vi "GetKingPosition.vi"(10 "Color":T1, 11 "Input Squares":T2[][](array[typedef])) -> (3 "Position":i32[](array[numeric]))   [LabVIEW 2019]
doc: "This VI searches chessboard in case of finding particular pieces"
uses:
  #typedef_SquareType.ctl
  #typedef_Color.ctl
  #typedef_Piece.ctl
  #typedef_PieceType.ctl
panel:
  out "?":u16[][](array[ring])
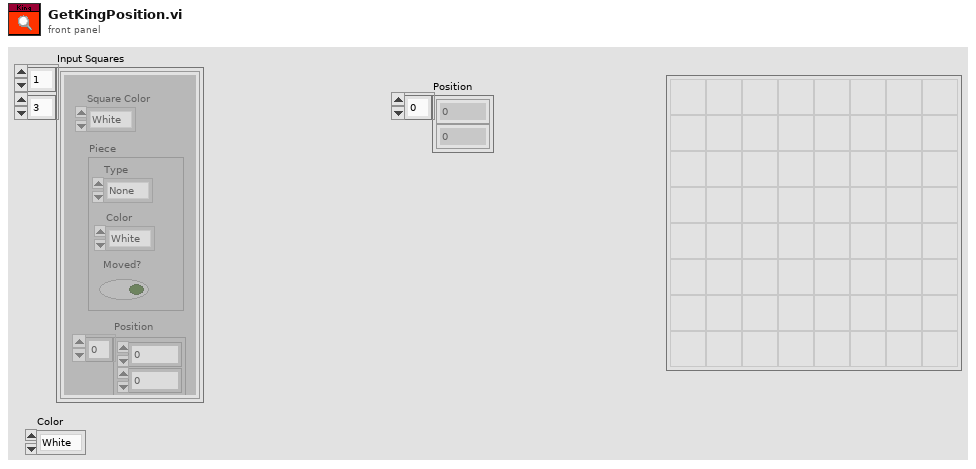
[diagram p1: front panel]
types:
  T1 = typedef "#typedef_Color.ctl" = enum16{"White", "Black"}
  T2 = typedef "#typedef_SquareType.ctl" = cluster{"Square Color":T1, "Position":i32[], "Piece":T3}
  T3 = typedef "#typedef_Piece.ctl" = cluster{"Type":T4, "Color":T1, "Moved?":bool}
  T4 = typedef "#typedef_PieceType.ctl" = enum16{"None", "Pawn", "Knight", "Bishop", "Rook", "Queen", "King"}
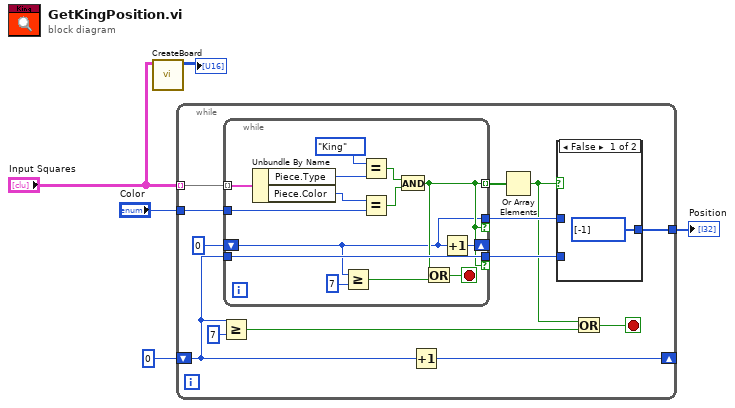
[diagram p0: block diagram]
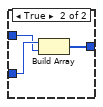
[diagram p2: hidden frame]
diagram:
  n1 = call "CreateBoard.vi"("Squares type"="Input Squares") -> ("Board"=→"?":u16[][])  [unwired: 10 in]
  n2 = while {
    tunnel: "Input Squares" -> [w18] mode=indexing
    tunnel: "Color" -> [w17]
    tunnel: [w13] -> w4
    shift-right: [w7] -> _
    shift-left: 0 -> [w6]
    stop <- w9 stop-if-true
    n3 = Greater Or Equal?(x=w6, y=7) -> (x >= y?=w10:bool)
    n4 = while {
      tunnel: w18 -> [w32] mode=indexing
      tunnel: w17 -> [w30]
      tunnel: w6 -> [w24]
      tunnel: [w24] -> w14 if=w21
      tunnel: [w19] -> w15 if=w21
      tunnel: [w21] -> w16 mode=indexing
      shift-right: [w20] -> _
      shift-left: 0 -> [w19]
      stop <- w25 stop-if-true
      n5 = Unbundle By Name(w32) -> ("Piece.Type"=w29:T4, "Piece.Color"=w31:T1)
      n6 = Greater Or Equal?(x=w19, y=7) -> (x >= y?=w22:bool)
      n7 = Equal?(x=#typedef_PieceType."King" ("Piece"), y=w29) -> (x = y?=w27:bool)
      n8 = Equal?(x=w31, y=w30) -> (x = y?=w26:bool)
      n9 = And(x=w27, y=w26) -> (x .and. y?=w21:bool)
      n10 = Or(x=w21, y=w22) -> (x .or. y?=w25:bool)
      n11 = Increment(x=w19) -> (x+1=w20:i32)
    }
    n12 = Increment(x=w6) -> (x+1=w7:i32)
    n13 = Or Array Elements(Boolean array=w16) -> (logical OR=w12:bool)
    n14 = case shown="False" w12 {
      tunnel: w15 -> [_ w34]
      tunnel: w14 -> [_ w35]
      tunnel: [i32[] [-1] w36] -> w13
      frame False {
      }
      frame True {
        n15 = Build Array(w35, w34) -> (w36:i32[])
      }
    }
    n16 = Or(x=w12, y=w10) -> (x .or. y?=w9:bool)
  }
  "Position" <- w4
